vi "Lab Panel V4.85.vi"() -> ()   [LabVIEW 2013] (continued)
                n1196 = case shown="True" w2167 {
                  tunnel: w2172 -> [_ w2176]
                  tunnel: w2166 -> [_ w2179]
                  frame False {
                  }
                  frame True {
                    n1197 = local read "SET LAB01-1"() -> (w2178:T5)
                    n1198 = local read "TDMS LAB01-1"() -> (w2175:refnum<k34>)
                    n1199 = Unbundle(w2176) -> ("CYCLE"=w2180:dbl)  [unwired: 2 out]
                    n1200 = Unbundle(w2178) -> ("T-RISE mins"=w2177:dbl)  [unwired: 4 out]
                    n1201 = Greater Or Equal?(x=w2180, y=w2179) -> (x >= y?=w2181:bool)
                    n1202 = case shown="True" w2181 {
                      tunnel: w2177 -> [w2184 _]
                      tunnel: w2176 -> [w2183 _]
                      tunnel: w2175 -> [w2182 _]
                      frame True {
                        n1203 = stacked-sequence {
                          tunnel: w2184 -> [w2187 _]
                          tunnel: w2183 -> [_ w2192]
                          tunnel: w2182 -> [w2185 _]
                          frame #0 {
                            n1204 = Build Array("T-RISE") -> (w2189:string[])
                            n1205 = Build Array(w2187) -> (w2188:dbl[])
                            n1206 = TDMS Write(0:w2185, 5:"TEST PASS", 7:w2189, 9:w2188) -> (15:w2191:errorcluster)  [unwired: 2 in, 3 out]
                            n1207 = local write "data file error"(w2191) -> ()
                          }
                          frame #1 {
                            n1208 = Bundle(cluster=w2192, "STATUS"="T-RISE PASS") -> (w2194:T4)  [unwired: 2 in]
                            n1209 = local write "RESULT LAB01-1"(TRUE) -> ()
                            n1210 = local write "DISP LAB01-1"(w2194) -> ()
                          }
                        }
                      }
                      frame False {
                      }
                    }
                  }
                }
              }
              frame #1 {
                # "LAB01-2"
                n1211 = Equal?(x=w2197, y=2) -> (x = y?=w2200:bool)
                n1212 = local read "DISP LAB01-2"() -> (w2202:T4)
                n1213 = Unbundle(w2202) -> ("STATUS"=w2203:string)  [unwired: 2 out]
                n1214 = Equal?(x=w2203, y="RUN") -> (x = y?=w2199:bool)
                n1215 = And(x=w2199, y=w2200) -> (x .and. y?=w2198:bool)
                n1216 = case shown="True" w2198 {
                  tunnel: w2202 -> [_ w2206]
                  tunnel: w2196 -> [_ w2209]
                  frame False {
                  }
                  frame True {
                    n1217 = local read "SET LAB01-2"() -> (w2208:T5)
                    n1218 = local read "TDMS LAB01-2"() -> (w2205:refnum<k34>)
                    n1219 = Unbundle(w2206) -> ("CYCLE"=w2210:dbl)  [unwired: 2 out]
                    n1220 = Unbundle(w2208) -> ("T-RISE mins"=w2207:dbl)  [unwired: 4 out]
                    n1221 = Greater Or Equal?(x=w2210, y=w2209) -> (x >= y?=w2211:bool)
                    n1222 = case shown="True" w2211 {
                      tunnel: w2207 -> [w2214 _]
                      tunnel: w2206 -> [w2213 _]
                      tunnel: w2205 -> [w2212 _]
                      frame True {
                        n1223 = stacked-sequence {
                          tunnel: w2214 -> [w2217 _]
                          tunnel: w2213 -> [_ w2222]
                          tunnel: w2212 -> [w2215 _]
                          frame #0 {
                            n1224 = Build Array("T-RISE") -> (w2219:string[])
                            n1225 = Build Array(w2217) -> (w2218:dbl[])
                            n1226 = TDMS Write(0:w2215, 5:"TEST PASS", 7:w2219, 9:w2218) -> (15:w2221:errorcluster)  [unwired: 2 in, 3 out]
                            n1227 = local write "data file error"(w2221) -> ()
                          }
                          frame #1 {
                            n1228 = Bundle(cluster=w2222, "STATUS"="T-RISE PASS") -> (w2224:T4)  [unwired: 2 in]
                            n1229 = local write "RESULT LAB01-2"(TRUE) -> ()
                            n1230 = local write "DISP LAB01-2"(w2224) -> ()
                          }
                        }
                      }
                      frame False {
                      }
                    }
                  }
                }
              }
              frame #2 {
                # "LAB02-1"
                n1231 = Equal?(x=w2227, y=2) -> (x = y?=w2230:bool)
                n1232 = local read "DISP LAB02-1"() -> (w2232:T4)
                n1233 = Unbundle(w2232) -> ("STATUS"=w2233:string)  [unwired: 2 out]
                n1234 = Equal?(x=w2233, y="RUN") -> (x = y?=w2229:bool)
                n1235 = And(x=w2229, y=w2230) -> (x .and. y?=w2228:bool)
                n1236 = case shown="True" w2228 {
                  tunnel: w2232 -> [_ w2236]
                  tunnel: w2226 -> [_ w2239]
                  frame False {
                  }
                  frame True {
                    n1237 = local read "SET LAB02-1"() -> (w2238:T5)
                    n1238 = local read "TDMS LAB02-1"() -> (w2235:refnum<k34>)
                    n1239 = Unbundle(w2236) -> ("CYCLE"=w2240:dbl)  [unwired: 2 out]
                    n1240 = Unbundle(w2238) -> ("T-RISE mins"=w2237:dbl)  [unwired: 4 out]
                    n1241 = Greater Or Equal?(x=w2240, y=w2239) -> (x >= y?=w2241:bool)
                    n1242 = case shown="True" w2241 {
                      tunnel: w2237 -> [w2244 _]
                      tunnel: w2236 -> [w2243 _]
                      tunnel: w2235 -> [w2242 _]
                      frame True {
                        n1243 = stacked-sequence {
                          tunnel: w2244 -> [w2247 _]
                          tunnel: w2243 -> [_ w2252]
                          tunnel: w2242 -> [w2245 _]
                          frame #0 {
                            n1244 = Build Array("T-RISE") -> (w2249:string[])
                            n1245 = Build Array(w2247) -> (w2248:dbl[])
                            n1246 = TDMS Write(0:w2245, 5:"TEST PASS", 7:w2249, 9:w2248) -> (15:w2251:errorcluster)  [unwired: 2 in, 3 out]
                            n1247 = local write "data file error"(w2251) -> ()
                          }
                          frame #1 {
                            n1248 = Bundle(cluster=w2252, "STATUS"="T-RISE PASS") -> (w2254:T4)  [unwired: 2 in]
                            n1249 = local write "RESULT LAB02-1"(TRUE) -> ()
                            n1250 = local write "DISP LAB02-1"(w2254) -> ()
                          }
                        }
                      }
                      frame False {
                      }
                    }
                  }
                }
              }
              frame #3 {
                # "LAB02-2"
                n1251 = Equal?(x=w2257, y=2) -> (x = y?=w2260:bool)
                n1252 = local read "DISP LAB02-2"() -> (w2262:T4)
                n1253 = Unbundle(w2262) -> ("STATUS"=w2263:string)  [unwired: 2 out]
                n1254 = Equal?(x=w2263, y="RUN") -> (x = y?=w2259:bool)
                n1255 = And(x=w2259, y=w2260) -> (x .and. y?=w2258:bool)
                n1256 = case shown="True" w2258 {
                  tunnel: w2262 -> [_ w2266]
                  tunnel: w2256 -> [_ w2269]
                  frame False {
                  }
                  frame True {
                    n1257 = local read "SET LAB02-2"() -> (w2268:T5)
                    n1258 = local read "TDMS LAB02-2"() -> (w2265:refnum<k34>)
                    n1259 = Unbundle(w2266) -> ("CYCLE"=w2270:dbl)  [unwired: 2 out]
                    n1260 = Unbundle(w2268) -> ("T-RISE mins"=w2267:dbl)  [unwired: 4 out]
                    n1261 = Greater Or Equal?(x=w2270, y=w2269) -> (x >= y?=w2271:bool)
                    n1262 = case shown="True" w2271 {
                      tunnel: w2267 -> [w2274 _]
                      tunnel: w2266 -> [w2273 _]
                      tunnel: w2265 -> [w2272 _]
                      frame True {
                        n1263 = stacked-sequence {
                          tunnel: w2274 -> [w2277 _]
                          tunnel: w2273 -> [_ w2282]
                          tunnel: w2272 -> [w2275 _]
                          frame #0 {
                            n1264 = Build Array("T-RISE") -> (w2279:string[])
                            n1265 = Build Array(w2277) -> (w2278:dbl[])
                            n1266 = TDMS Write(0:w2275, 5:"TEST PASS", 7:w2279, 9:w2278) -> (15:w2281:errorcluster)  [unwired: 2 in, 3 out]
                            n1267 = local write "data file error"(w2281) -> ()
                          }
                          frame #1 {
                            n1268 = Bundle(cluster=w2282, "STATUS"="T-RISE PASS") -> (w2284:T4)  [unwired: 2 in]
                            n1269 = local write "RESULT LAB02-2"(TRUE) -> ()
                            n1270 = local write "DISP LAB02-2"(w2284) -> ()
                          }
                        }
                      }
                      frame False {
                      }
                    }
                  }
                }
              }
              frame #4 {
                # "LAB03-1"
                n1271 = Equal?(x=w2287, y=2) -> (x = y?=w2290:bool)
                n1272 = local read "DISP LAB03-1"() -> (w2292:T4)
                n1273 = Unbundle(w2292) -> ("STATUS"=w2293:string)  [unwired: 2 out]
                n1274 = Equal?(x=w2293, y="RUN") -> (x = y?=w2289:bool)
                n1275 = And(x=w2289, y=w2290) -> (x .and. y?=w2288:bool)
                n1276 = case shown="True" w2288 {
                  tunnel: w2292 -> [_ w2296]
                  tunnel: w2286 -> [_ w2299]
                  frame False {
                  }
                  frame True {
                    n1277 = local read "SET LAB03-1"() -> (w2298:T5)
                    n1278 = local read "TDMS LAB03-1"() -> (w2295:refnum<k34>)
                    n1279 = Unbundle(w2296) -> ("CYCLE"=w2300:dbl)  [unwired: 2 out]
                    n1280 = Unbundle(w2298) -> ("T-RISE mins"=w2297:dbl)  [unwired: 4 out]
                    n1281 = Greater Or Equal?(x=w2300, y=w2299) -> (x >= y?=w2301:bool)
                    n1282 = case shown="True" w2301 {
                      tunnel: w2297 -> [w2304 _]
                      tunnel: w2296 -> [w2303 _]
                      tunnel: w2295 -> [w2302 _]
                      frame True {
                        n1283 = stacked-sequence {
                          tunnel: w2304 -> [w2307 _]
                          tunnel: w2303 -> [_ w2312]
                          tunnel: w2302 -> [w2305 _]
                          frame #0 {
                            n1284 = Build Array("T-RISE") -> (w2309:string[])
                            n1285 = Build Array(w2307) -> (w2308:dbl[])
                            n1286 = TDMS Write(0:w2305, 5:"TEST PASS", 7:w2309, 9:w2308) -> (15:w2311:errorcluster)  [unwired: 2 in, 3 out]
                            n1287 = local write "data file error"(w2311) -> ()
                          }
                          frame #1 {
                            n1288 = Bundle(cluster=w2312, "STATUS"="T-RISE PASS") -> (w2314:T4)  [unwired: 2 in]
                            n1289 = local write "RESULT LAB03-1"(TRUE) -> ()
                            n1290 = local write "DISP LAB03-1"(w2314) -> ()
                          }
                        }
                      }
                      frame False {
                      }
                    }
                  }
                }
              }
              frame #5 {
                # "LAB03-2"
                n1291 = Equal?(x=w2317, y=2) -> (x = y?=w2320:bool)
                n1292 = local read "DISP LAB03-2"() -> (w2322:T4)
                n1293 = Unbundle(w2322) -> ("STATUS"=w2323:string)  [unwired: 2 out]
                n1294 = Equal?(x=w2323, y="RUN") -> (x = y?=w2319:bool)
                n1295 = And(x=w2319, y=w2320) -> (x .and. y?=w2318:bool)
                n1296 = case shown="True" w2318 {
                  tunnel: w2322 -> [_ w2326]
                  tunnel: w2316 -> [_ w2329]
                  frame False {
                  }
                  frame True {
                    n1297 = local read "SET LAB03-2"() -> (w2328:T5)
                    n1298 = local read "TDMS LAB03-2"() -> (w2325:refnum<k34>)
                    n1299 = Unbundle(w2326) -> ("CYCLE"=w2330:dbl)  [unwired: 2 out]
                    n1300 = Unbundle(w2328) -> ("T-RISE mins"=w2327:dbl)  [unwired: 4 out]
                    n1301 = Greater Or Equal?(x=w2330, y=w2329) -> (x >= y?=w2331:bool)
                    n1302 = case shown="True" w2331 {
                      tunnel: w2327 -> [w2334 _]
                      tunnel: w2326 -> [w2333 _]
                      tunnel: w2325 -> [w2332 _]
                      frame True {
                        n1303 = stacked-sequence {
                          tunnel: w2334 -> [w2337 _]
                          tunnel: w2333 -> [_ w2342]
                          tunnel: w2332 -> [w2335 _]
                          frame #0 {
                            n1304 = Build Array("T-RISE") -> (w2339:string[])
                            n1305 = Build Array(w2337) -> (w2338:dbl[])
                            n1306 = TDMS Write(0:w2335, 5:"TEST PASS", 7:w2339, 9:w2338) -> (15:w2341:errorcluster)  [unwired: 2 in, 3 out]
                            n1307 = local write "data file error"(w2341) -> ()
                          }
                          frame #1 {
                            n1308 = Bundle(cluster=w2342, "STATUS"="T-RISE PASS") -> (w2344:T4)  [unwired: 2 in]
                            n1309 = local write "RESULT LAB03-2"(TRUE) -> ()
                            n1310 = local write "DISP LAB03-2"(w2344) -> ()
                          }
                        }
                      }
                      frame False {
                      }
                    }
                  }
                }
              }
              frame #6 {
                # "LAB04-1"
                n1311 = Equal?(x=w2347, y=2) -> (x = y?=w2350:bool)
                n1312 = local read "DISP LAB04-1"() -> (w2352:T4)
                n1313 = Unbundle(w2352) -> ("STATUS"=w2353:string)  [unwired: 2 out]
                n1314 = Equal?(x=w2353, y="RUN") -> (x = y?=w2349:bool)
                n1315 = And(x=w2349, y=w2350) -> (x .and. y?=w2348:bool)
                n1316 = case shown="True" w2348 {
                  tunnel: w2352 -> [_ w2356]
                  tunnel: w2346 -> [_ w2359]
                  frame False {
                  }
                  frame True {
                    n1317 = local read "SET LAB04-1"() -> (w2358:T5)
                    n1318 = local read "TDMS LAB04-1"() -> (w2355:refnum<k34>)
                    n1319 = Unbundle(w2356) -> ("CYCLE"=w2360:dbl)  [unwired: 2 out]
                    n1320 = Unbundle(w2358) -> ("T-RISE mins"=w2357:dbl)  [unwired: 4 out]
                    n1321 = Greater Or Equal?(x=w2360, y=w2359) -> (x >= y?=w2361:bool)
                    n1322 = case shown="True" w2361 {
                      tunnel: w2357 -> [w2364 _]
                      tunnel: w2356 -> [w2363 _]
                      tunnel: w2355 -> [w2362 _]
                      frame True {
                        n1323 = stacked-sequence {
                          tunnel: w2364 -> [w2367 _]
                          tunnel: w2363 -> [_ w2372]
                          tunnel: w2362 -> [w2365 _]
                          frame #0 {
                            n1324 = Build Array("T-RISE") -> (w2369:string[])
                            n1325 = Build Array(w2367) -> (w2368:dbl[])
                            n1326 = TDMS Write(0:w2365, 5:"TEST PASS", 7:w2369, 9:w2368) -> (15:w2371:errorcluster)  [unwired: 2 in, 3 out]
                            n1327 = local write "data file error"(w2371) -> ()
                          }
                          frame #1 {
                            n1328 = Bundle(cluster=w2372, "STATUS"="T-RISE PASS") -> (w2374:T4)  [unwired: 2 in]
                            n1329 = local write "RESULT LAB04-1"(TRUE) -> ()
                            n1330 = local write "DISP LAB04-1"(w2374) -> ()
                          }
                        }
                      }
                      frame False {
                      }
                    }
                  }
                }
              }
              frame #7 {
                # "LAB04-2"
                n1331 = Equal?(x=w2377, y=2) -> (x = y?=w2380:bool)
                n1332 = local read "DISP LAB04-2"() -> (w2382:T4)
                n1333 = Unbundle(w2382) -> ("STATUS"=w2383:string)  [unwired: 2 out]
                n1334 = Equal?(x=w2383, y="RUN") -> (x = y?=w2379:bool)
                n1335 = And(x=w2379, y=w2380) -> (x .and. y?=w2378:bool)
                n1336 = case shown="True" w2378 {
                  tunnel: w2382 -> [_ w2386]
                  tunnel: w2376 -> [_ w2389]
                  frame False {
                  }
                  frame True {
                    n1337 = local read "SET LAB04-2"() -> (w2388:T5)
                    n1338 = local read "TDMS LAB04-2"() -> (w2385:refnum<k34>)
                    n1339 = Unbundle(w2386) -> ("CYCLE"=w2390:dbl)  [unwired: 2 out]
                    n1340 = Unbundle(w2388) -> ("T-RISE mins"=w2387:dbl)  [unwired: 4 out]
                    n1341 = Greater Or Equal?(x=w2390, y=w2389) -> (x >= y?=w2391:bool)
                    n1342 = case shown="True" w2391 {
                      tunnel: w2387 -> [w2394 _]
                      tunnel: w2386 -> [w2393 _]
                      tunnel: w2385 -> [w2392 _]
                      frame True {
                        n1343 = stacked-sequence {
                          tunnel: w2394 -> [w2397 _]
                          tunnel: w2393 -> [_ w2402]
                          tunnel: w2392 -> [w2395 _]
                          frame #0 {
                            n1344 = Build Array("T-RISE") -> (w2399:string[])
                            n1345 = Build Array(w2397) -> (w2398:dbl[])
                            n1346 = TDMS Write(0:w2395, 5:"TEST PASS", 7:w2399, 9:w2398) -> (15:w2401:errorcluster)  [unwired: 2 in, 3 out]
                            n1347 = local write "data file error"(w2401) -> ()
                          }
                          frame #1 {
                            n1348 = Bundle(cluster=w2402, "STATUS"="T-RISE PASS") -> (w2404:T4)  [unwired: 2 in]
                            n1349 = local write "RESULT LAB04-2"(TRUE) -> ()
                            n1350 = local write "DISP LAB04-2"(w2404) -> ()
                          }
                        }
                      }
                      frame False {
                      }
                    }
                  }
                }
              }
              frame #8 {
                # "LAB05-1"
                n1351 = Equal?(x=w2407, y=2) -> (x = y?=w2410:bool)
                n1352 = local read "DISP LAB05-1"() -> (w2412:T4)
                n1353 = Unbundle(w2412) -> ("STATUS"=w2413:string)  [unwired: 2 out]
                n1354 = Equal?(x=w2413, y="RUN") -> (x = y?=w2409:bool)
                n1355 = And(x=w2409, y=w2410) -> (x .and. y?=w2408:bool)
                n1356 = case shown="True" w2408 {
                  tunnel: w2412 -> [_ w2416]
                  tunnel: w2406 -> [_ w2419]
                  frame False {
                  }
                  frame True {
                    n1357 = local read "SET LAB05-1"() -> (w2418:T5)
                    n1358 = local read "TDMS LAB05-1"() -> (w2415:refnum<k34>)
                    n1359 = Unbundle(w2416) -> ("CYCLE"=w2420:dbl)  [unwired: 2 out]
                    n1360 = Unbundle(w2418) -> ("T-RISE mins"=w2417:dbl)  [unwired: 4 out]
                    n1361 = Greater Or Equal?(x=w2420, y=w2419) -> (x >= y?=w2421:bool)
                    n1362 = case shown="True" w2421 {
                      tunnel: w2417 -> [w2424 _]
                      tunnel: w2416 -> [w2423 _]
                      tunnel: w2415 -> [w2422 _]
                      frame True {
                        n1363 = stacked-sequence {
                          tunnel: w2424 -> [w2427 _]
                          tunnel: w2423 -> [_ w2432]
                          tunnel: w2422 -> [w2425 _]
                          frame #0 {
                            n1364 = Build Array("T-RISE") -> (w2429:string[])
                            n1365 = Build Array(w2427) -> (w2428:dbl[])
                            n1366 = TDMS Write(0:w2425, 5:"TEST PASS", 7:w2429, 9:w2428) -> (15:w2431:errorcluster)  [unwired: 2 in, 3 out]
                            n1367 = local write "data file error"(w2431) -> ()
                          }
                          frame #1 {
                            n1368 = Bundle(cluster=w2432, "STATUS"="T-RISE PASS") -> (w2434:T4)  [unwired: 2 in]
                            n1369 = local write "RESULT LAB05-1"(TRUE) -> ()
                            n1370 = local write "DISP LAB05-1"(w2434) -> ()
                          }
                        }
                      }
                      frame False {
                      }
                    }
                  }
                }
              }
              frame #9 {
                # "LAB05-2"
                n1371 = Equal?(x=w2437, y=2) -> (x = y?=w2440:bool)
                n1372 = local read "DISP LAB05-2"() -> (w2442:T4)
                n1373 = Unbundle(w2442) -> ("STATUS"=w2443:string)  [unwired: 2 out]
                n1374 = Equal?(x=w2443, y="RUN") -> (x = y?=w2439:bool)
                n1375 = And(x=w2439, y=w2440) -> (x .and. y?=w2438:bool)
                n1376 = case shown="True" w2438 {
                  tunnel: w2442 -> [_ w2446]
                  tunnel: w2436 -> [_ w2449]
                  frame False {
                  }
                  frame True {
                    n1377 = local read "SET LAB05-2"() -> (w2448:T5)
                    n1378 = local read "TDMS LAB05-2"() -> (w2445:refnum<k34>)
                    n1379 = Unbundle(w2446) -> ("CYCLE"=w2450:dbl)  [unwired: 2 out]
                    n1380 = Unbundle(w2448) -> ("T-RISE mins"=w2447:dbl)  [unwired: 4 out]
                    n1381 = Greater Or Equal?(x=w2450, y=w2449) -> (x >= y?=w2451:bool)
                    n1382 = case shown="True" w2451 {
                      tunnel: w2447 -> [w2454 _]
                      tunnel: w2446 -> [w2453 _]
                      tunnel: w2445 -> [w2452 _]
                      frame True {
                        n1383 = stacked-sequence {
                          tunnel: w2454 -> [w2457 _]
                          tunnel: w2453 -> [_ w2462]
                          tunnel: w2452 -> [w2455 _]
                          frame #0 {
                            n1384 = Build Array("T-RISE") -> (w2459:string[])
                            n1385 = Build Array(w2457) -> (w2458:dbl[])
                            n1386 = TDMS Write(0:w2455, 5:"TEST PASS", 7:w2459, 9:w2458) -> (15:w2461:errorcluster)  [unwired: 2 in, 3 out]
                            n1387 = local write "data file error"(w2461) -> ()
                          }
                          frame #1 {
                            n1388 = Bundle(cluster=w2462, "STATUS"="T-RISE PASS") -> (w2464:T4)  [unwired: 2 in]
                            n1389 = local write "RESULT LAB05-2"(TRUE) -> ()
                            n1390 = local write "DISP LAB05-2"(w2464) -> ()
                          }
                        }
                      }
                      frame False {
                      }
                    }
                  }
                }
              }
            }
          }
          frame #6 {
            # "end test & close test files"
            n1391 = local read "MAIL SETTINGS"() -> (w2470:T6)
            n1392 = Unbundle(w2470) -> ("OUT SERVER ADDRESS"=w2469:string, "FROM ACCOUNT"=w2468:string)  [unwired: 5 out]
            n1393 = stacked-sequence {
              tunnel: w2480 -> [_ _ _ _ _ _ _ _ _ _]
              tunnel: w2481 -> [_ _ _ _ _ _ _ _ _ _]
              tunnel: w2479 -> [_ _ _ _ _ _ _ _ _ _]
              tunnel: w2478 -> [_ _ _ _ _ _ _ _ _ _]
              tunnel: w2477 -> [_ _ _ _ _ _ _ _ _ _]
              tunnel: w2476 -> [_ _ _ _ _ _ _ _ _ _]
              tunnel: w2475 -> [_ _ _ _ _ _ _ _ _ _]
              tunnel: w2474 -> [_ _ _ _ _ _ _ _ _ _]
              tunnel: w2473 -> [_ _ _ _ _ _ _ _ _ _]
              tunnel: w2472 -> [_ _ _ _ _ _ _ _ _ _]
              tunnel: w2469 -> [w2485 w2537 w2585 w2632 w2679 w2726 w2773 w2820 w2867 w2914]
              tunnel: w2468 -> [w2484 w2536 w2584 w2631 w2678 w2725 w2772 w2819 w2866 w2913]
              tunnel: "Test File To" -> [w2483 w2535 w2583 w2630 w2677 w2724 w2771 w2818 w2865 w2912]
              tunnel: "Mail Test Fail" -> [w2482 w2534 w2582 w2629 w2676 w2723 w2770 w2817 w2864 w2911]
              frame #0 {
                # "LAB01-1"
                n1394 = local read "DISP LAB01-1"() -> (w2489:T4)
                n1395 = local read "run lab01-1"() -> (w2486:bool)
                n1396 = local read "TDMS LAB01-1"() -> (w2487:refnum<k34>)
                n1397 = Unbundle(w2489) -> ("CYCLE"=w2490:dbl, "STATUS"=w2488:string)  [unwired: 1 out]
                n1398 = case shown="True" w2486 {
                  tunnel: w2490 -> [_ w2496]
                  tunnel: w2489 -> [_ w2498]
                  tunnel: w2488 -> [_ w2495]
                  tunnel: w2487 -> [_ w2497]
                  tunnel: w2485 -> [_ w2494]
                  tunnel: w2484 -> [_ w2493]
                  tunnel: w2483 -> [_ w2492]
                  tunnel: w2482 -> [_ w2491]
                  frame False {
                  }
                  frame True {
                    n1399 = Not Equal?(x=w2495, y="RUN") -> (x != y?=w2499:bool)
                    n1400 = Greater?(x=w2496, y=2.0) -> (0:w2501:bool)
                    n1401 = And(x=w2501, y=w2499) -> (x .and. y?=w2500:bool)
                    n1402 = case shown="True" w2500 {
                      tunnel: w2498 -> [_ w2511]
                      tunnel: w2497 -> [_ w2510]
                      tunnel: w2496 -> [_ w2509]
                      tunnel: w2495 -> [_ w2508]
                      tunnel: w2494 -> [_ w2507]
                      tunnel: w2493 -> [_ w2506]
                      tunnel: w2492 -> [_ w2505]
                      tunnel: w2491 -> [_ w2504]
                      frame False {
                      }
                      frame True {
                        n1403 = stacked-sequence {
                          tunnel: w2511 -> [w2515 _ _]
                          tunnel: w2510 -> [_ w2517 _]
                          tunnel: w2509 -> [_ _ _]
                          tunnel: w2508 -> [_ _ w2523]
                          tunnel: w2507 -> [_ _ w2522]
                          tunnel: w2506 -> [_ _ w2521]
                          tunnel: w2505 -> [_ _ w2520]
                          tunnel: w2504 -> [_ _ w2519]
                          frame #0 {
                            w2512 = FALSE
                            n1404 = local write "mail control"("END") -> ()
                            n1405 = Bundle(cluster=w2515) -> (w2514:T4)  [unwired: 3 in]
                            n1406 = local write "DISP LAB01-1"(w2514) -> ()
                            n1407 = local write "O/I  LAB01-1"(w2512) -> ()
                            n1408 = local write "run lab01-1"(w2512) -> ()
                            n1409 = local write "RUN LAB01-1"(w2512) -> ()
                          }
                          frame #1 {
                            n1410 = TDMS Close(11:w2517) -> (0:w2516:errorcluster)  [unwired: 1 in, 1 out]
                            n1411 = local write "data file error"(w2516) -> ()
                          }
                          frame #2 {
                            n1412 = stacked-sequence {
                              tunnel: "LAB01-1" -> [w2525 w2527 _]
                              tunnel: w2523 -> [_ w2533 _]
                              tunnel: w2522 -> [_ w2532 _]
                              tunnel: w2521 -> [_ w2531 _]
                              tunnel: w2520 -> [_ w2530 _]
                              tunnel: w2519 -> [_ w2529 _]
                              frame #0 {
                                n1413 = call "sub vi - defrag tdms v1.vi"("panel id"=w2525) -> ("error out"=w2524:errorcluster)  [unwired: 10 in]
                                n1414 = local write "data file error"(w2524) -> ()
                              }
                              frame #1 {
                                n1415 = Bundle("STATUS"=w2533, "OUT SERVER ADDRESS"=w2532, "FROM ACCOUNT"=w2531, "Test File To"=w2530, "Mail Test Fail"=w2529) -> (w2526:T23)  [unwired: 1 in]
                                n1416 = call "Save data file to network drive v3.vi"("Input Cluster"=w2526, "panel id"=w2527) -> ("network file save error"=w2528:errorcluster)  [unwired: 8 in, 1 out]
                                n1417 = local write "data file error"(w2528) -> ()
                              }
                              frame #2 {
                              }
                            }
                          }
                        }
                      }
                    }
                  }
                }
              }
              frame #1 {
                # "LAB01-2"
                n1418 = local read "run lab01-2"() -> (w2538:bool)
                n1419 = case shown="True" w2538 {
                  tunnel: w2537 -> [_ w2542]
                  tunnel: w2536 -> [_ w2541]
                  tunnel: w2535 -> [_ w2540]
                  tunnel: w2534 -> [_ w2539]
                  frame False {
                  }
                  frame True {
                    n1420 = local read "DISP LAB01-2"() -> (w2550:T4)
                    n1421 = local read "TDMS LAB01-2"() -> (w2549:refnum<k34>)
                    n1422 = Unbundle(w2550) -> ("CYCLE"=w2544:dbl, "STATUS"=w2543:string)  [unwired: 1 out]
                    n1423 = Not Equal?(x=w2543, y="RUN") -> (x != y?=w2546:bool)
                    n1424 = Greater?(x=w2544, y=2.0) -> (0:w2547:bool)
                    n1425 = And(x=w2547, y=w2546) -> (x .and. y?=w2545:bool)
                    n1426 = case shown="True" w2545 {
                      tunnel: w2550 -> [_ w2559]
                      tunnel: w2549 -> [_ w2558]
                      tunnel: w2544 -> [_ w2557]
                      tunnel: w2543 -> [_ w2556]
                      tunnel: w2542 -> [_ w2555]
                      tunnel: w2541 -> [_ w2554]
                      tunnel: w2540 -> [_ w2553]
                      tunnel: w2539 -> [_ w2552]
                      frame False {
                      }
                      frame True {
                        n1427 = stacked-sequence {
                          tunnel: w2559 -> [w2562 _ _]
                          tunnel: w2558 -> [_ w2564 _]
                          tunnel: w2557 -> [_ _ _]
                          tunnel: w2556 -> [_ _ w2570]
                          tunnel: w2555 -> [_ _ w2569]
                          tunnel: w2554 -> [_ _ w2568]
                          tunnel: w2553 -> [_ _ w2567]
                          tunnel: w2552 -> [_ _ w2566]
                          frame #0 {
                            w2560 = FALSE
                            n1428 = local write "mail control"("END") -> ()
                            n1429 = Bundle(cluster=w2562) -> (w2563:T4)  [unwired: 3 in]
                            n1430 = local write "RUN LAB01-2"(w2560) -> ()
                            n1431 = local write "run lab01-2"(w2560) -> ()
                            n1432 = local write "O/I  LAB01-2"(w2560) -> ()
                            n1433 = local write "DISP LAB01-2"(w2563) -> ()
                          }
                          frame #1 {
                            n1434 = TDMS Close(11:w2564) -> (0:w2565:errorcluster)  [unwired: 1 in, 1 out]
                            n1435 = local write "data file error"(w2565) -> ()
                          }
                          frame #2 {
                            n1436 = stacked-sequence {
                              tunnel: "LAB01-2" -> [w2573 w2574]
                              tunnel: w2570 -> [_ w2579]
                              tunnel: w2569 -> [_ w2578]
                              tunnel: w2568 -> [_ w2577]
                              tunnel: w2567 -> [_ w2576]
                              tunnel: w2566 -> [_ w2575]
                              frame #0 {
                                n1437 = call "sub vi - defrag tdms v1.vi"("panel id"=w2573) -> ("error out"=w2572:errorcluster)  [unwired: 10 in]
                                n1438 = local write "data file error"(w2572) -> ()
                              }
                              frame #1 {
                                n1439 = Bundle("STATUS"=w2579, "OUT SERVER ADDRESS"=w2578, "FROM ACCOUNT"=w2577, "Test File To"=w2576, "Mail Test Fail"=w2575) -> (w2581:T23)  [unwired: 1 in]
                                n1440 = call "Save data file to network drive v3.vi"("Input Cluster"=w2581, "panel id"=w2574) -> ("network file save error"=w2580:errorcluster)  [unwired: 8 in, 1 out]
                                n1441 = local write "data file error"(w2580) -> ()
                              }
                            }
                          }
                        }
                      }
                    }
                  }
                }
              }
              frame #2 {
                # "LAB02-1"
                n1442 = local read "run lab02-1"() -> (w2586:bool)
                n1443 = case shown="True" w2586 {
                  tunnel: w2585 -> [_ w2590]
                  tunnel: w2584 -> [_ w2589]
                  tunnel: w2583 -> [_ w2588]
                  tunnel: w2582 -> [_ w2587]
                  frame False {
                  }
                  frame True {
                    n1444 = local read "DISP LAB02-1"() -> (w2598:T4)
                    n1445 = Unbundle(w2598) -> ("CYCLE"=w2594:dbl, "STATUS"=w2591:string)  [unwired: 1 out]
                    n1446 = local read "TDMS LAB02-1"() -> (w2597:refnum<k34>)
                    n1447 = Not Equal?(x=w2591, y="RUN") -> (x != y?=w2593:bool)
                    n1448 = Greater?(x=w2594, y=2.0) -> (0:w2595:bool)
                    n1449 = And(x=w2595, y=w2593) -> (x .and. y?=w2592:bool)
                    n1450 = case shown="True" w2592 {
                      tunnel: w2598 -> [_ w2606]
                      tunnel: w2597 -> [_ w2605]
                      tunnel: w2591 -> [_ w2604]
                      tunnel: w2590 -> [_ w2603]
                      tunnel: w2589 -> [_ w2602]
                      tunnel: w2588 -> [_ w2601]
                      tunnel: w2587 -> [_ w2600]
                      frame False {
                      }
                      frame True {
                        n1451 = stacked-sequence {
                          tunnel: w2606 -> [w2609 _ _]
                          tunnel: w2605 -> [_ w2611 _]
                          tunnel: w2604 -> [_ _ w2617]
                          tunnel: w2603 -> [_ _ w2616]
                          tunnel: w2602 -> [_ _ w2615]
                          tunnel: w2601 -> [_ _ w2614]
                          tunnel: w2600 -> [_ _ w2613]
                          frame #0 {
                            w2607 = FALSE
                            n1452 = local write "mail control"("END") -> ()
                            n1453 = Bundle(cluster=w2609) -> (w2610:T4)  [unwired: 3 in]
                            n1454 = local write "O/I  LAB02-1"(w2607) -> ()
                            n1455 = local write "RUN LAB02-1"(w2607) -> ()
                            n1456 = local write "run lab02-1"(w2607) -> ()
                            n1457 = local write "DISP LAB02-1"(w2610) -> ()
                          }
                          frame #1 {
                            n1458 = TDMS Close(11:w2611) -> (0:w2612:errorcluster)  [unwired: 1 in, 1 out]
                            n1459 = local write "data file error"(w2612) -> ()
                          }
                          frame #2 {
                            n1460 = stacked-sequence {
                              tunnel: "LAB02-1" -> [w2620 w2627]
                              tunnel: w2617 -> [_ w2625]
                              tunnel: w2616 -> [_ w2624]
                              tunnel: w2615 -> [_ w2623]
                              tunnel: w2614 -> [_ w2622]
                              tunnel: w2613 -> [_ w2621]
                              frame #0 {
                                n1461 = call "sub vi - defrag tdms v1.vi"("panel id"=w2620) -> ("error out"=w2619:errorcluster)  [unwired: 10 in]
                                n1462 = local write "data file error"(w2619) -> ()
                              }
                              frame #1 {
                                n1463 = Bundle("STATUS"=w2625, "OUT SERVER ADDRESS"=w2624, "FROM ACCOUNT"=w2623, "Test File To"=w2622, "Mail Test Fail"=w2621) -> (w2626:T23)  [unwired: 1 in]
                                n1464 = call "Save data file to network drive v3.vi"("Input Cluster"=w2626, "panel id"=w2627) -> ("network file save error"=w2628:errorcluster)  [unwired: 8 in, 1 out]
                                n1465 = local write "data file error"(w2628) -> ()
                              }
                            }
                          }
                        }
                      }
                    }
                  }
                }
              }
              frame #3 {
                # "LAB02-2"
                n1466 = local read "run lab02-2"() -> (w2633:bool)
                n1467 = case shown="True" w2633 {
                  tunnel: w2632 -> [_ w2637]
                  tunnel: w2631 -> [_ w2636]
                  tunnel: w2630 -> [_ w2635]
                  tunnel: w2629 -> [_ w2634]
                  frame False {
                  }
                  frame True {
                    n1468 = local read "DISP LAB02-2"() -> (w2645:T4)
                    n1469 = local read "TDMS LAB02-2"() -> (w2644:refnum<k34>)
                    n1470 = Unbundle(w2645) -> ("CYCLE"=w2641:dbl, "STATUS"=w2638:string)  [unwired: 1 out]
                    n1471 = Not Equal?(x=w2638, y="RUN") -> (x != y?=w2640:bool)
                    n1472 = Greater?(x=w2641, y=2.0) -> (0:w2642:bool)
                    n1473 = And(x=w2642, y=w2640) -> (x .and. y?=w2639:bool)
                    n1474 = case shown="True" w2639 {
                      tunnel: w2645 -> [_ w2653]
                      tunnel: w2644 -> [_ w2652]
                      tunnel: w2638 -> [_ w2651]
                      tunnel: w2637 -> [_ w2650]
                      tunnel: w2636 -> [_ w2649]
                      tunnel: w2635 -> [_ w2648]
                      tunnel: w2634 -> [_ w2647]
                      frame False {
                      }
                      frame True {
                        n1475 = stacked-sequence {
                          tunnel: w2653 -> [w2656 _ _]
                          tunnel: w2652 -> [_ w2658 _]
                          tunnel: w2651 -> [_ _ w2664]
                          tunnel: w2650 -> [_ _ w2663]
                          tunnel: w2649 -> [_ _ w2662]
                          tunnel: w2648 -> [_ _ w2661]
                          tunnel: w2647 -> [_ _ w2660]
                          frame #0 {
                            w2654 = FALSE
                            n1476 = local write "mail control"("END") -> ()
                            n1477 = Bundle(cluster=w2656) -> (w2657:T4)  [unwired: 3 in]
                            n1478 = local write "O/I  LAB02-2"(w2654) -> ()
                            n1479 = local write "run lab02-2"(w2654) -> ()
                            n1480 = local write "RUN LAB02-2"(w2654) -> ()
                            n1481 = local write "DISP LAB02-2"(w2657) -> ()
                          }
                          frame #1 {
                            n1482 = TDMS Close(11:w2658) -> (0:w2659:errorcluster)  [unwired: 1 in, 1 out]
                            n1483 = local write "data file error"(w2659) -> ()
                          }
                          frame #2 {
                            n1484 = stacked-sequence {
                              tunnel: "LAB02-2" -> [w2667 w2673]
                              tunnel: w2664 -> [_ w2672]
                              tunnel: w2663 -> [_ w2671]
                              tunnel: w2662 -> [_ w2670]
                              tunnel: w2661 -> [_ w2669]
                              tunnel: w2660 -> [_ w2668]
                              frame #0 {
                                n1485 = call "sub vi - defrag tdms v1.vi"("panel id"=w2667) -> ("error out"=w2666:errorcluster)  [unwired: 10 in]
                                n1486 = local write "data file error"(w2666) -> ()
                              }
                              frame #1 {
                                n1487 = Bundle("STATUS"=w2672, "OUT SERVER ADDRESS"=w2671, "FROM ACCOUNT"=w2670, "Test File To"=w2669, "Mail Test Fail"=w2668) -> (w2675:T23)  [unwired: 1 in]
                                n1488 = call "Save data file to network drive v3.vi"("Input Cluster"=w2675, "panel id"=w2673) -> ("network file save error"=w2674:errorcluster)  [unwired: 8 in, 1 out]
                                n1489 = local write "data file error"(w2674) -> ()
                              }
                            }
                          }
                        }
                      }
                    }
                  }
                }
              }
              frame #4 {
                # "LAB03-1"
                n1490 = local read "run lab03-1"() -> (w2680:bool)
                n1491 = case shown="True" w2680 {
                  tunnel: w2679 -> [_ w2684]
                  tunnel: w2678 -> [_ w2683]
                  tunnel: w2677 -> [_ w2682]
                  tunnel: w2676 -> [_ w2681]
                  frame False {
                  }
                  frame True {
                    n1492 = local read "DISP LAB03-1"() -> (w2692:T4)
                    n1493 = local read "TDMS LAB03-1"() -> (w2691:refnum<k34>)
                    n1494 = Unbundle(w2692) -> ("CYCLE"=w2688:dbl, "STATUS"=w2685:string)  [unwired: 1 out]
                    n1495 = Not Equal?(x=w2685, y="RUN") -> (x != y?=w2687:bool)
                    n1496 = Greater?(x=w2688, y=2.0) -> (0:w2689:bool)
                    n1497 = And(x=w2689, y=w2687) -> (x .and. y?=w2686:bool)
                    n1498 = case shown="True" w2686 {
                      tunnel: w2692 -> [_ w2700]
                      tunnel: w2691 -> [_ w2699]
                      tunnel: w2685 -> [_ w2698]
                      tunnel: w2684 -> [_ w2697]
                      tunnel: w2683 -> [_ w2696]
                      tunnel: w2682 -> [_ w2695]
                      tunnel: w2681 -> [_ w2694]
                      frame False {
                      }
                      frame True {
                        n1499 = stacked-sequence {
                          tunnel: w2700 -> [w2703 _ _]
                          tunnel: w2699 -> [_ w2705 _]
                          tunnel: w2698 -> [_ _ w2711]
                          tunnel: w2697 -> [_ _ w2710]
                          tunnel: w2696 -> [_ _ w2709]
                          tunnel: w2695 -> [_ _ w2708]
                          tunnel: w2694 -> [_ _ w2707]
                          frame #0 {
                            w2701 = FALSE
                            n1500 = local write "mail control"("END") -> ()
                            n1501 = Bundle(cluster=w2703) -> (w2704:T4)  [unwired: 3 in]
                            n1502 = local write "O/I  LAB03-1"(w2701) -> ()
                            n1503 = local write "run lab03-1"(w2701) -> ()
                            n1504 = local write "RUN LAB03-1"(w2701) -> ()
                            n1505 = local write "DISP LAB03-1"(w2704) -> ()
                          }
                          frame #1 {
                            n1506 = TDMS Close(11:w2705) -> (0:w2706:errorcluster)  [unwired: 1 in, 1 out]
                            n1507 = local write "data file error"(w2706) -> ()
                          }
                          frame #2 {
                            n1508 = stacked-sequence {
                              tunnel: "LAB03-1" -> [w2714 w2720]
                              tunnel: w2711 -> [_ w2719]
                              tunnel: w2710 -> [_ w2718]
                              tunnel: w2709 -> [_ w2717]
                              tunnel: w2708 -> [_ w2716]
                              tunnel: w2707 -> [_ w2715]
                              frame #0 {
                                n1509 = call "sub vi - defrag tdms v1.vi"("panel id"=w2714) -> ("error out"=w2713:errorcluster)  [unwired: 10 in]
                                n1510 = local write "data file error"(w2713) -> ()
                              }
                              frame #1 {
                                n1511 = Bundle("STATUS"=w2719, "OUT SERVER ADDRESS"=w2718, "FROM ACCOUNT"=w2717, "Test File To"=w2716, "Mail Test Fail"=w2715) -> (w2722:T23)  [unwired: 1 in]
                                n1512 = call "Save data file to network drive v3.vi"("Input Cluster"=w2722, "panel id"=w2720) -> ("network file save error"=w2721:errorcluster)  [unwired: 8 in, 1 out]
                                n1513 = local write "data file error"(w2721) -> ()
                              }
                            }
                          }
                        }
                      }
                    }
                  }
                }
              }
              frame #5 {
                # "LAB03-2"
                n1514 = local read "run lab03-2"() -> (w2727:bool)
                n1515 = case shown="True" w2727 {
                  tunnel: w2726 -> [_ w2731]
                  tunnel: w2725 -> [_ w2730]
                  tunnel: w2724 -> [_ w2729]
                  tunnel: w2723 -> [_ w2728]
                  frame False {
                  }
                  frame True {
                    n1516 = local read "DISP LAB03-2"() -> (w2739:T4)
                    n1517 = Unbundle(w2739) -> ("CYCLE"=w2735:dbl, "STATUS"=w2732:string)  [unwired: 1 out]
                    n1518 = local read "TDMS LAB03-2"() -> (w2738:refnum<k34>)
                    n1519 = Not Equal?(x=w2732, y="RUN") -> (x != y?=w2734:bool)
                    n1520 = Greater?(x=w2735, y=2.0) -> (0:w2736:bool)
                    n1521 = And(x=w2736, y=w2734) -> (x .and. y?=w2733:bool)
                    n1522 = case shown="True" w2733 {
                      tunnel: w2739 -> [_ w2747]
                      tunnel: w2738 -> [_ w2746]
                      tunnel: w2732 -> [_ w2745]
                      tunnel: w2731 -> [_ w2744]
                      tunnel: w2730 -> [_ w2743]
                      tunnel: w2729 -> [_ w2742]
                      tunnel: w2728 -> [_ w2741]
                      frame False {
                      }
                      frame True {
                        n1523 = stacked-sequence {
                          tunnel: w2747 -> [w2750 _ _]
                          tunnel: w2746 -> [_ w2752 _]
                          tunnel: w2745 -> [_ _ w2758]
                          tunnel: w2744 -> [_ _ w2757]
                          tunnel: w2743 -> [_ _ w2756]
                          tunnel: w2742 -> [_ _ w2755]
                          tunnel: w2741 -> [_ _ w2754]
                          frame #0 {
                            w2748 = FALSE
                            n1524 = local write "mail control"("END") -> ()
                            n1525 = Bundle(cluster=w2750) -> (w2751:T4)  [unwired: 3 in]
                            n1526 = local write "RUN LAB03-2"(w2748) -> ()
                            n1527 = local write "O/I  LAB03-2"(w2748) -> ()
                            n1528 = local write "DISP LAB03-2"(w2751) -> ()
